vi "Timing Measurement Page - Multi FPGA.vi"(8 "error in (no error)":errorcluster, 11 "Node Ptr":T2 format="%.0x") -> (0 "error out":errorcluster)   [LabVIEW 2015, in "Engine Simulation Toolkit System Explorer.lvlib"]
uses:
  Engine Simulation Toolkit System Explorer.lvlib
  <vilib>/NI Veristand/Custom Device API/Custom Device Item Ref.ctl
  Polarity.ctl
  Shared/Properties.vi
  <vilib>/NI Veristand/Custom Device API/Get Item Property (String).vi
  <vilib>/NI Veristand/Custom Device API/Get Item Property (U16).vi
  Shared/Constants and GUIDs.vi
  <vilib>/NI Veristand/Custom Device API/Custom Device API.lvlib
  Shared/Engine Simulation Toolkit Shared.lvlib
panel:
  out "Polarity":T1
  out "Window":string
  out "Name in bitfile":string
  in  "Name":string
  in  "Header 2":cluster{"Section Name":string}={"Section Name"="Event Captures"}
  in  "remove cap":bool
  in  "add cap":bool
  in  "Capture listbox":i32[](listbox) caption="Available Event Captures"
  in  "Header":cluster{"Section Name":string}={"Section Name"="Measurement"}
  # "Timing measurement settings are configured on the parent page"
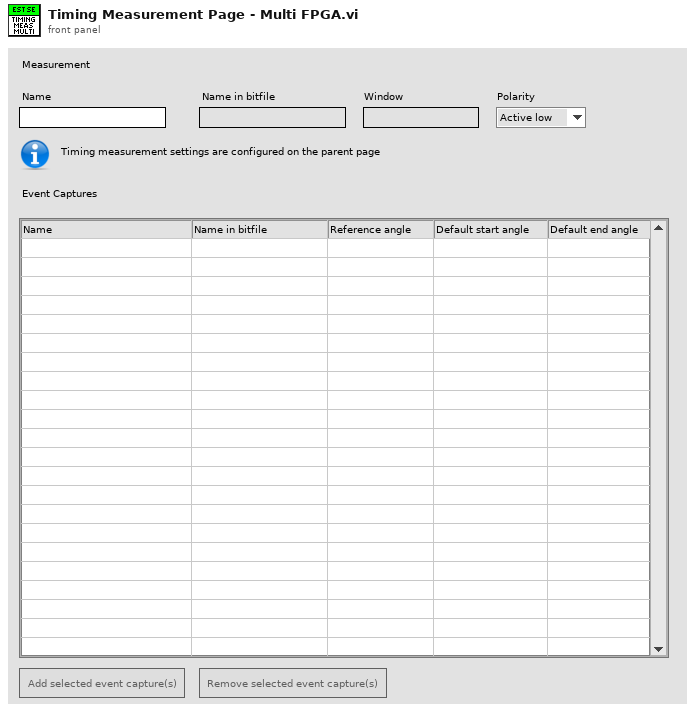
[diagram p1: front panel]
types:
  T1 = typedef "Engine Simulation Toolkit System Explorer.lvlib/Polarity.ctl" = enum16{"Active low", "Active high"}
  T2 = typedef "Custom Device API.lvlib/Custom Device Item Ref.ctl" = u64
  T3 = typedef "Custom Device API.lvlib/Custom Device Item Info.ctl" = cluster{"Name":string, "Is Channel":bool, "GUID":string, "Is Waveform":bool}
  T4 = typedef "Engine Simulation Toolkit System Explorer.lvlib/Event Timing Capture.ctl" = cluster{"Name":string, "Bitfile name":string, "Reference angle":dbl, "Default start":dbl, "Default end":dbl, "Ref Select":T5}
  T5 = typedef "Engine Simulation Toolkit System Explorer.lvlib/Event Reference Angle Selection.ctl" = enum16{"From window", "Custom"}
  T6 = typedef "Custom Device API.lvlib/Custom Device Commands.ctl" = enum16{"Default", "Item renamed", "Shutdown", "Dynamic button pressed"}
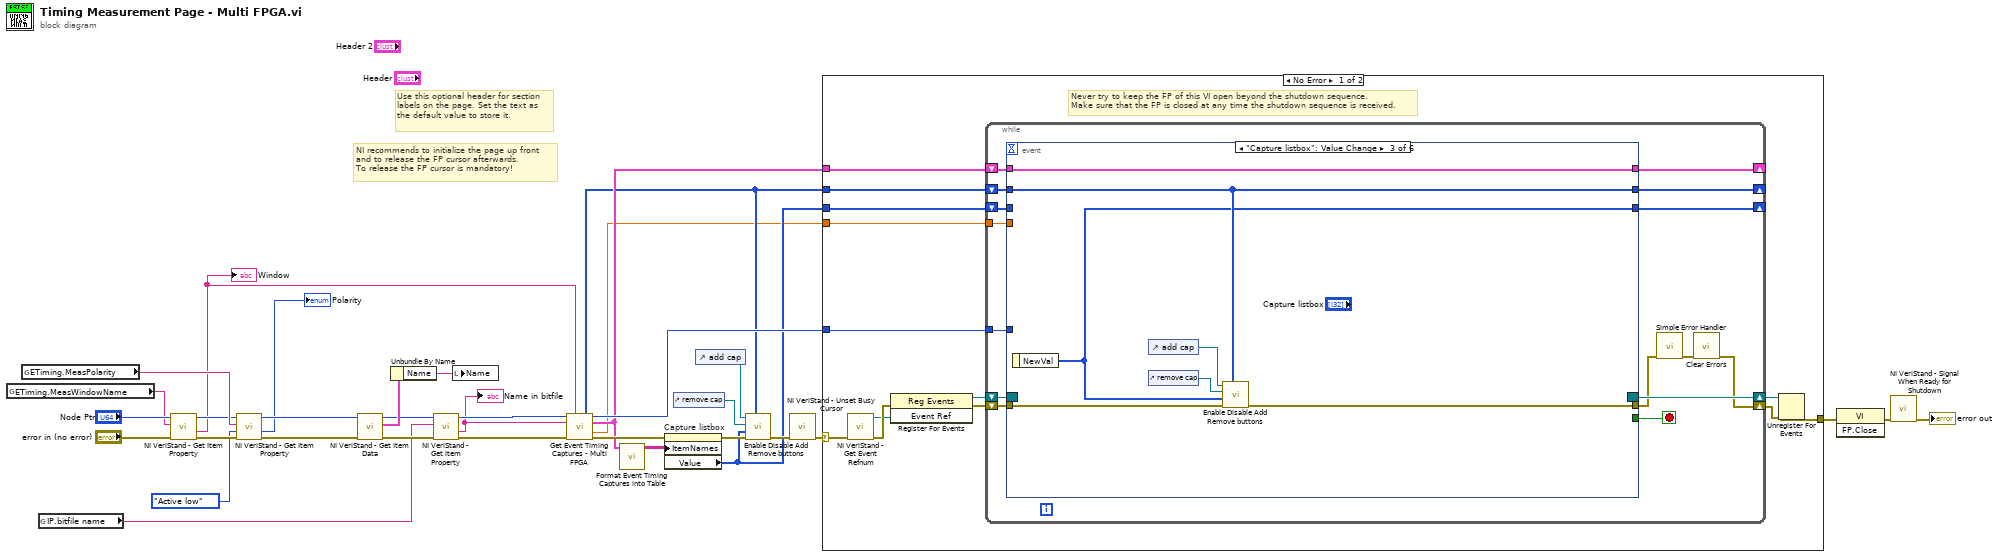
[diagram p0: block diagram]
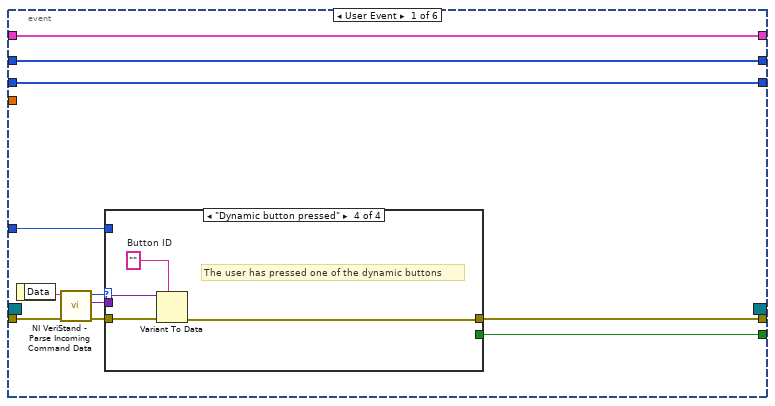
[diagram p2: hidden frame]
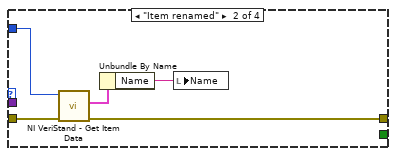
[diagram p4: hidden frame]
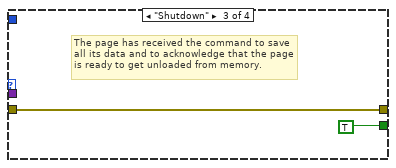
[diagram p5: hidden frame]
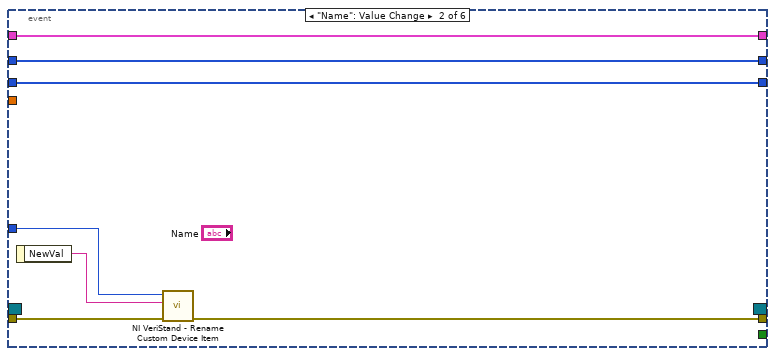
[diagram p6: hidden frame]
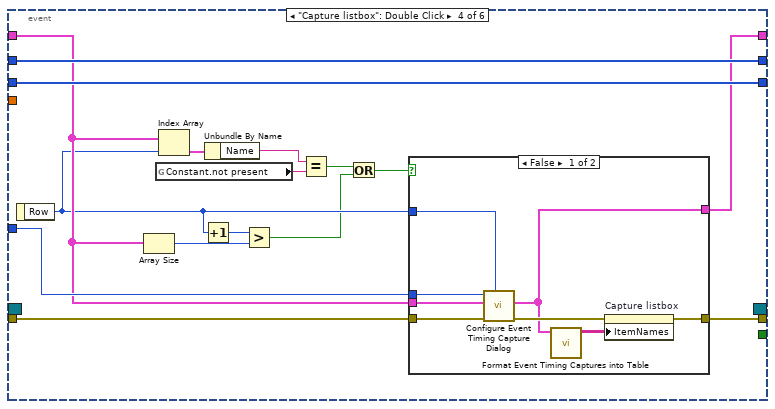
[diagram p7: hidden frame]
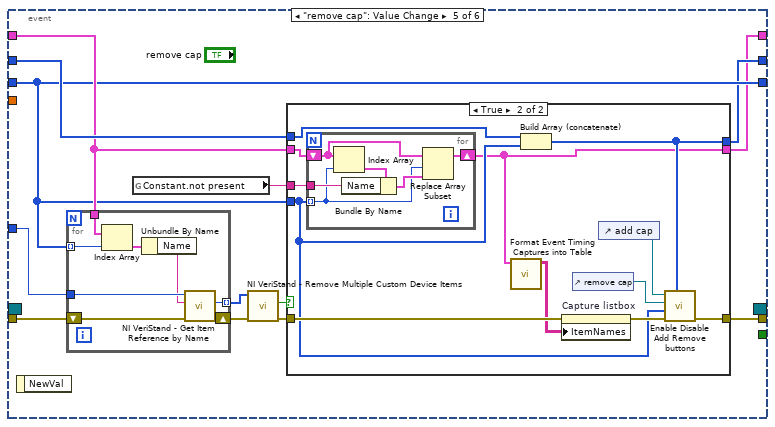
[diagram p9: hidden frame]
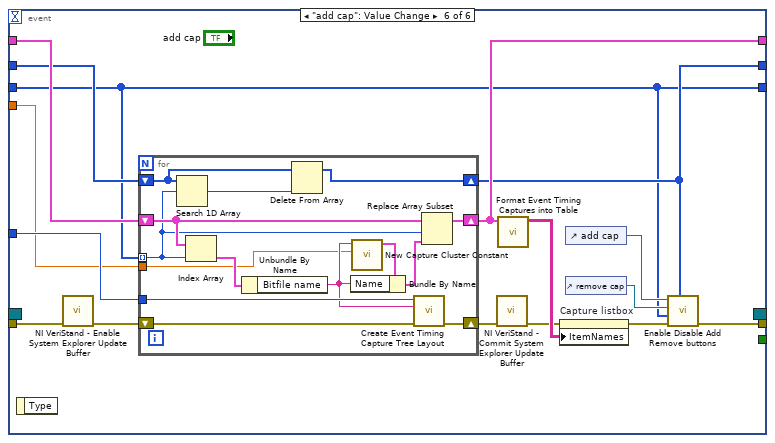
[diagram p11: hidden frame]
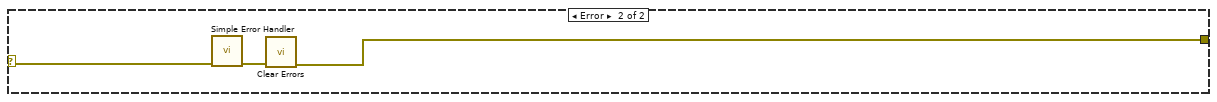
[diagram p12: hidden frame]
diagram:
  # "Use this optional header for section labels on the page. Set the text as the default value to store it."
  # "NI recommends to initialize the page up front\nand to release the FP cursor afterwards.\nTo release the FP cursor is mandatory!"
  n1 = global read "Properties.vi" "ETiming.MeasWindowName"() -> (w26:string)
  n2 = global read "Properties.vi" "ETiming.MeasPolarity"() -> (w25:string)
  n3 = global read "Properties.vi" "IP.bitfile name"() -> (w13:string)
  n4 = call-poly <vilib>:"NI VeriStand - Get Item Property.vi"("error in (no error)"="error in (no error)", "Property Name"=w26, "Item Ref in"="Node Ptr") -> ("error out"=w21:errorcluster, "Value"=w2:string, "Item Ref out"=w24:T2)  [unwired: 5 in, 1 out]
  "Window" <- w2
  n5 = call-poly <vilib>:"NI VeriStand - Get Item Property.vi"("error in (no error)"=w21, "Default Value"=Polarity."Active low" ("Polarity"), "Property Name"=w25, "Item Ref in"=w24) -> ("error out"=w22:errorcluster, "Value"=→"Polarity":u16, "Item Ref out"=w23:T2)  [unwired: 4 in, 1 out]
  n6 = call <vilib>:"NI VeriStand - Get Item Data.vi"("error in (no error)"=w22, "Item Ref in"=w23) -> ("error out"=w19:errorcluster, "Item Info"=w18:T3, "Item Ref out"=w15:T2)  [unwired: 6 in, 1 out]
  n7 = Unbundle By Name(w18) -> ("Name"=w17:string)
  n8 = call-poly <vilib>:"NI VeriStand - Get Item Property.vi"("error in (no error)"=w19, "Property Name"=w13, "Item Ref in"=w15) -> ("error out"=w16:errorcluster, "Value"=w11:string, "Item Ref out"=w14:T2)  [unwired: 5 in, 1 out]
  "Name in bitfile" <- w11
  n9 = local write "Name"(w17) -> ()
  n10 = call "Get Event Timing Captures - Multi FPGA.vi"("Item Ref in"=w14, "Window"=w2, "Timing measurement"=w11, "error in (no error)"=w16) -> ("not present indexes"=w4:i32[], "Item Ref out"=w29:T2, "captures"=w9:T4[], "Window reference angle"=w1:dbl, "error out"=w28:errorcluster)  [unwired: 3 in, 4 out]
  n11 = call "Format Event Timing Captures into Table.vi"("Captures"=w9) -> ("Table"=w10:string[][])  [unwired: 10 in]
  n12 = property on="Capture listbox" class="MCListbox (strict)"(error in=w28, "ItemNames"=w10) -> (error out=w6:errorcluster, "Value"=w3:i32[])  [unwired: 1 in, 1 out]
  n13 = control-ref of="remove cap"() -> (w8:refnum<vi>)
  n14 = control-ref of="add cap"() -> (w7:refnum<vi>)
  n15 = call "Enable Disable Add Remove buttons.vi"("not present item indexes"=w4, "error in (no error)"=w6, "selected items"=w3, "remove button"=w8, "add button"=w7) -> ("error out"=w5:errorcluster)  [unwired: 6 in]
  n16 = call <vilib>:"NI VeriStand - Unset Busy Cursor.vi"("error in (no error)"=w5) -> ("error out"=w30:errorcluster)  [unwired: 10 out]
  n17 = case shown="No Error" w30 {
    selector: w30 -> [w39 w200]
    tunnel: [w44 w198] -> w34
    tunnel: w29 -> [w40 _]
    tunnel: w4 -> [w38 _]
    tunnel: w9 -> [w37 _]
    tunnel: w3 -> [w36 _]
    tunnel: w1 -> [w35 _]
    frame No Error {
      # "Never try to keep the FP of this VI open beyond the shutdown sequence.\nMake sure that the FP is closed at any time the shutdown sequence is received."
      n18 = call <vilib>:"NI VeriStand - Get Event Refnum.vi"("error in (no error)"=w39) -> ("error out"=w47:errorcluster, "Event Ref"=w43:refnum<user-event>)  [unwired: 9 out]
      n19 = register-events(error in=w47, w43) -> (reference out=w41:refnum<event-registration>, error out=w42:errorcluster)  [unwired: 1 in]
      n20 = while {
        tunnel: w40 -> [w58]
        shift-right: [w55] -> w45
        shift-left: w42 -> [w61]
        shift-right: [w62] -> w46
        shift-left: w41 -> [w60]
        shift-right: [w51] -> _
        shift-left: w38 -> [w54]
        shift-right: [w52] -> _
        shift-left: w37 -> [w53]
        shift-right: [w50] -> _
        shift-left: w36 -> [w49]
        tunnel: w35 -> [w48]
        stop <- w59 stop-if-true
        n21 = event shown="[2] \"Capture listbox\": Value Change" {
          selector: w60 -> [_ _ _ _ _ _]
          dyn-events: [_ _ _ _ _ _] -> w62
          timeout: _ -> [_ _ _ _ _ _]
          tunnel: w61 -> [w73 w92 w98 w110 w133 w176]
          tunnel: [w69 _ _ _ _ _] -> w59
          tunnel: [w68 w91 w97 w109 w132 w175] -> w57
          tunnel: w58 -> [w67 w90 _ w108 w126 w174]
          tunnel: w54 -> [w64 w87 w94 w115 w131 w171]
          tunnel: w53 -> [w65 w88 w99 w102 w130 w173]
          tunnel: [w65 w88 w99 w107 w127 w172] -> w52
          tunnel: [w64 w87 w94 w115 w128 w170] -> w51
          tunnel: [w63 w86 w93 w114 w129 w169] -> w50
          tunnel: w49 -> [w63 w86 _ w114 w129 w169]
          tunnel: w48 -> [_ _ _ _ _ w168]
          event User Event {
            n22 = event-data() -> ("Data"=w72:string)  [unwired: 1 out]
            n23 = call <vilib>:"NI VeriStand - Parse Incoming Command Data.vi"("error in (no error)"=w73, "Incoming data"=w72) -> ("error out"=w71:errorcluster, "Outgoing data"=w66:variant, "Action"=w70:T6)  [unwired: 7 out]
            n24 = case shown="\"Dynamic button pressed\"" w70 {
              tunnel: w71 -> [w74 w79 w80 w85]
              tunnel: [_ _ TRUE _] -> w69
              tunnel: [w74 w75 w80 w82] -> w68
              tunnel: w67 -> [_ w78 _ _]
              tunnel: w66 -> [_ _ _ w84]
              frame "Default", Default {
              }
              frame "Item renamed" {
                n25 = call <vilib>:"NI VeriStand - Get Item Data.vi"("error in (no error)"=w79, "Item Ref in"=w78) -> ("error out"=w75:errorcluster, "Item Info"=w76:T3)  [unwired: 6 in, 2 out]
                n26 = Unbundle By Name(w76) -> ("Name"=w77:string)
                n27 = local write "Name"(w77) -> ()
              }
              frame "Shutdown" {
                # "The page has received the command to save all its data and to acknowledge that the page is ready to get unloaded from memory."
              }
              frame "Dynamic button pressed" {
                w83 = ""  # Button ID
                # "The user has pressed one of the dynamic buttons"
                n28 = Variant To Data(error in=w85, type=w83, Variant=w84) -> (error out=w82:errorcluster)  [unwired: 1 out]
              }
            }
          }
          event "Name": Value Change {
            n29 = event-data() -> ("NewVal"=w89:string)  [unwired: 1 out]
            n30 = call <vilib>:"NI VeriStand - Rename Custom Device Item.vi"("error in (no error)"=w92, "New Name"=w89, "Item Ref in"=w90) -> ("error out"=w91:errorcluster)  [unwired: 6 in, 2 out]
          }
          event "Capture listbox": Value Change {
            n31 = event-data() -> ("NewVal"=w93:i32[])  [unwired: 1 out]
            n32 = control-ref of="add cap"() -> (w96:refnum<vi>)
            n33 = control-ref of="remove cap"() -> (w95:refnum<vi>)
            n34 = call "Enable Disable Add Remove buttons.vi"("not present item indexes"=w94, "error in (no error)"=w98, "selected items"=w93, "remove button"=w95, "add button"=w96) -> ("error out"=w97:errorcluster)  [unwired: 6 in]
          }
          event "Capture listbox": Double Click {
            n35 = event-data() -> ("Row"=w101:i32)  [unwired: 1 out]
            n36 = Array Size(array=w102) -> (size(s)=w104:i32)
            n37 = global read "Constants and GUIDs.vi" "Constant.not present"() -> (w112:string)
            n38 = Index Array(array=w102, index=w101) -> (element=w111:T4)
            n39 = Increment(x=w101) -> (x+1=w103:i32)
            n40 = Unbundle By Name(w111) -> ("Name"=w113:string)
            n41 = Greater?(x=w103, y=w104) -> (0:w100:bool)
            n42 = Equal?(x=w113, y=w112) -> (x = y?=w106:bool)
            n43 = Or(x=w106, y=w100) -> (x .or. y?=w105:bool)
            n44 = case shown="False" w105 {
              tunnel: w110 -> [w123 w124]
              tunnel: [w118 w124] -> w109
              tunnel: w101 -> [w122 _]
              tunnel: w108 -> [w121 _]
              tunnel: w102 -> [w117 w125]
              tunnel: [w116 w125] -> w107
              frame False {
                n45 = call "Configure Event Timing Capture Dialog.vi"("capture to be edited"=w122, "error in (no error)"=w123, "captures in"=w117, "Item Ref in"=w121) -> ("error out"=w119:errorcluster, "captures out"=w116:T4[])  [unwired: 5 in, 1 out]
                n46 = call "Format Event Timing Captures into Table.vi"("Captures"=w116) -> ("Table"=w120:string[][])  [unwired: 10 in]
                n47 = property on="Capture listbox" class="MCListbox (strict)"(error in=w119, "ItemNames"=w120) -> (error out=w118:errorcluster)  [unwired: 1 in, 1 out]
              }
              frame True {
              }
            }
          }
          event "remove cap": Value Change {
            n48 = event-data() -> ()  [unwired: 2 out]
            n49 = for {
              tunnel: w129 -> [w162] mode=indexing
              tunnel: w130 -> [w163]
              tunnel: w126 -> [w166]
              tunnel: [w164] -> w135 mode=indexing
              shift-right: [w165] -> w134
              shift-left: w133 -> [w167]
              n50 = Index Array(array=w163, index=w162) -> (element=w161:T4)
              n51 = Unbundle By Name(w161) -> ("Name"=w160:string)
              n52 = call <vilib>:"NI VeriStand - Get Item Reference by Name.vi"("error in (no error)"=w167, "Item Name"=w160, "Parent Ref in"=w166) -> ("error out"=w165:errorcluster, "Item Ref"=w164:T2)  [unwired: 5 in, 2 out]
            }
            n53 = global read "Constants and GUIDs.vi" "Constant.not present"() -> (w138:string)
            n54 = call <vilib>:"NI VeriStand - Remove Multiple Custom Device Items.vi"("error in (no error)"=w134, "Item Refs in"=w135) -> ("error out"=w136:errorcluster, "Deleted?"=w137:bool)  [unwired: 8 in]
            n55 = case shown="True" w137 {
              tunnel: [w140 w152] -> w132
              tunnel: w136 -> [w140 w151]
              tunnel: w129 -> [_ w147]
              tunnel: w130 -> [w141 w150]
              tunnel: w138 -> [_ w149]
              tunnel: [w141 w143] -> w127
              tunnel: w131 -> [w139 w148]
              tunnel: [w139 w146] -> w128
              frame False {
              }
              frame True {
                n56 = for {
                  tunnel: w147 -> [w154] mode=indexing
                  shift-right: [w156] -> w143
                  shift-left: w150 -> [w157]
                  tunnel: w149 -> [w158]
                  n57 = Index Array(array=w157, index=w154) -> (element=w159:T4)
                  n58 = Bundle By Name(cluster=w159, "Name"=w158) -> (w155:T4)
                  n59 = Replace Array Subset(array=w157, new element=w155, index=w154) -> (w156:T4[])
                }
                n60 = call "Format Event Timing Captures into Table.vi"("Captures"=w143) -> ("Table"=w142:string[][])  [unwired: 10 in]
                n61 = Build Array (concatenate)(w148, w147) -> (w146:i32[])
                n62 = property on="Capture listbox" class="MCListbox (strict)"(error in=w151, "ItemNames"=w142) -> (error out=w153:errorcluster)  [unwired: 1 in, 1 out]
                n63 = control-ref of="remove cap"() -> (w144:refnum<vi>)
                n64 = control-ref of="add cap"() -> (w145:refnum<vi>)
                n65 = call "Enable Disable Add Remove buttons.vi"("not present item indexes"=w146, "error in (no error)"=w153, "selected items"=w147, "remove button"=w144, "add button"=w145) -> ("error out"=w152:errorcluster)  [unwired: 6 in]
              }
            }
          }
          event "add cap": Value Change {
            n66 = event-data() -> ()  [unwired: 2 out]
            n67 = call <vilib>:"NI VeriStand - Enable System Explorer Update Buffer.vi"("error in (no error)"=w176) -> ("error out"=w178:errorcluster)  [unwired: 10 in]
            n68 = for {
              tunnel: w174 -> [w195]
              shift-right: [w196] -> w180
              shift-left: w178 -> [w197]
              tunnel: w169 -> [w192] mode=indexing
              shift-right: [w193] -> w172
              shift-left: w173 -> [w194]
              shift-right: [w189] -> w170
              shift-left: w171 -> [w191]
              tunnel: w168 -> [w184]
              n69 = Search 1D Array(1D array=w191, element=w192) -> (index of element=w190:i32)  [unwired: 1 in]
              n70 = Index Array(array=w194, index=w192) -> (element=w188:T4)
              n71 = Unbundle By Name(w188) -> ("Bitfile name"=w185:string)
              n72 = Delete From Array(array=w191, index=w190) -> (array with subset deleted=w189:i32[])  [unwired: 1 in, 1 out]
              n73 = call "New Capture Cluster Constant.vi"("Window ref angle"=w184, "Bitfile name"=w185) -> ("Capture"=w186:T4)  [unwired: 9 in]
              n74 = Bundle By Name(cluster=w186, "Name"=w185) -> (w187:T4)
              n75 = call "Create Event Timing Capture Tree Layout.vi"("error in (no error)"=w197, "capture name"=w185, "Section Ptr"=w195) -> ("error out"=w196:errorcluster)  [unwired: 7 in, 1 out]
              n76 = Replace Array Subset(array=w194, new element=w187, index=w192) -> (w193:T4[])
            }
            n77 = call <vilib>:"NI VeriStand - Commit System Explorer Update Buffer.vi"("error in (no error)"=w180) -> ("error out"=w177:errorcluster)  [unwired: 10 in]
            n78 = call "Format Event Timing Captures into Table.vi"("Captures"=w172) -> ("Table"=w179:string[][])  [unwired: 10 in]
            n79 = property on="Capture listbox" class="MCListbox (strict)"(error in=w177, "ItemNames"=w179) -> (error out=w183:errorcluster)  [unwired: 1 in, 1 out]
            n80 = control-ref of="add cap"() -> (w182:refnum<vi>)
            n81 = control-ref of="remove cap"() -> (w181:refnum<vi>)
            n82 = call "Enable Disable Add Remove buttons.vi"("not present item indexes"=w170, "error in (no error)"=w183, "selected items"=w169, "remove button"=w181, "add button"=w182) -> ("error out"=w175:errorcluster)  [unwired: 6 in]
          }
        }
        n83 = call <vilib>:"Simple Error Handler.vi"("error in (no error)"=w57) -> ("error out"=w56:errorcluster)  [unwired: 1 in, 7 out]
        n84 = call <vilib>:"Clear Errors.vi"("error in (no error)"=w56) -> ("error out"=w55:errorcluster)  [unwired: 1 in, 5 out]
      }
      n85 = Unregister For Events(event registration refnum=w46, error in=w45) -> (error out=w44:errorcluster)
    }
    frame Error {
      n86 = call <vilib>:"Simple Error Handler.vi"("error in (no error)"=w200) -> ("error out"=w199:errorcluster)  [unwired: 1 in, 7 out]
      n87 = call <vilib>:"Clear Errors.vi"("error in (no error)"=w199) -> ("error out"=w198:errorcluster)  [unwired: 1 in, 5 out]
    }
  }
  n88 = invoke class="VI" method="FP.Close"(error in=w34) -> (error out=w33:errorcluster)  [unwired: 2 in, 2 out]
  n89 = call <vilib>:"NI VeriStand - Signal When Ready for Shutdown.vi"("error in (no error)"=w33) -> ("error out"=→"error out":errorcluster)  [unwired: 10 out]
